vi "表格和打印表格.vi"() -> ()   [LabVIEW 2023]
panel:
  out "new picture":picture
  in  "Multicolumn Listbox":i32(listbox)
  # "表格以及打印表格"
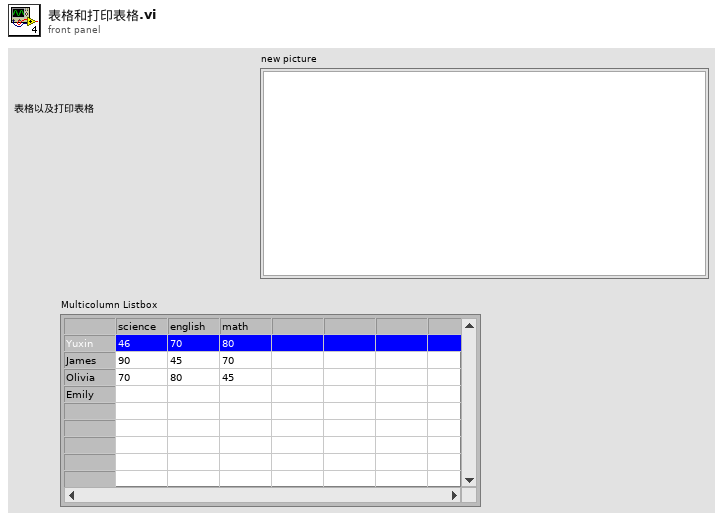
[diagram p1: front panel]
types:
  T1 = typedef "imagedata.ctl" = cluster{"image type":i32, "image depth":i32, "image":u8[], "mask":u8[], "colors":u32[], "Rectangle":cluster{"left":i16, "top":i16, "right":i16, "bottom":i16}}
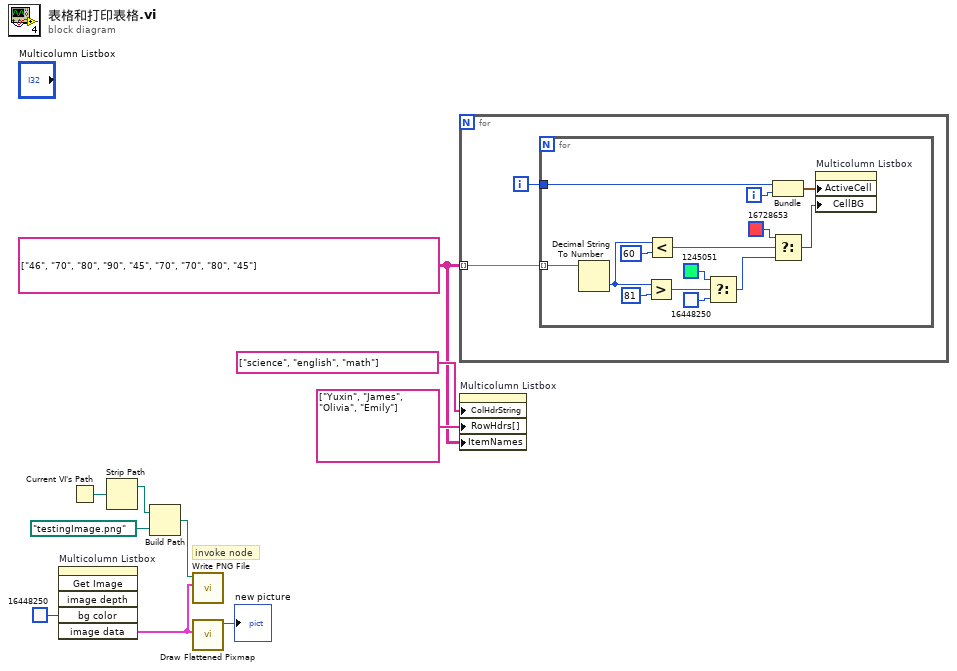
[diagram p0: block diagram]
diagram:
  w8 = string[][] [["46", "70", "80"], ["90", "45", "70"], ["70", "80", "45"]]
  # "invoke node"
  n1 = invoke on="Multicolumn Listbox" class="MCListbox (strict)" method="Get Image"("bg color"=u32 16448250) -> ("image data"=w5:T1)  [unwired: 5 in, 5 out]
  n2 = Current VI's Path() -> (path=w4:path)
  n3 = Strip Path(path=w4) -> (stripped path=w3:path)  [unwired: 1 out]
  n4 = Build Path(base path=w3, name or relative path=path "testingImage.png") -> (appended path=w1:path)
  n5 = call <vilib>:"Write PNG File.vi"("image data"=w5, "path to PNG file"=w1) -> ()  [unwired: 8 in, 2 out]
  n6 = call <vilib>:"Draw Flattened Pixmap.vi"("image data"=w5) -> ("new picture"=→"new picture":picture)  [unwired: 8 in]
  n7 = for {
    tunnel: w8 -> [w11] mode=indexing
    i -> [w12]
    n8 = for {
      tunnel: w12 -> [w26]
      tunnel: w11 -> [w23] mode=indexing
      i -> [w25]
      n9 = Decimal String To Number(string=w23) -> (number=w17:i32)  [unwired: 2 in, 1 out]
      n10 = Greater?(x=w17, y=81) -> (0:w15:bool)
      n11 = Less?(x=w17, y=60) -> (x < y?=w21:bool)
      n12 = Select(t=u32 1245051, s=w15, f=u32 16448250) -> (s? t:f=w18:u32)
      n13 = Bundle(w26, w25) -> (w24:cluster{i32, i32})  [unwired: 1 in]
      n14 = Select(t=u32 16728653, s=w21, f=w18) -> (s? t:f=w19:u32)
      n15 = property on="Multicolumn Listbox" class="MCListbox (strict)"("ActiveCell"=w24, "CellBG"=w19) -> ()  [unwired: 2 in, 2 out]
    }
  }
  n16 = property on="Multicolumn Listbox" class="MCListbox (strict)"("ColHdrString"=string[] ["science", "english", "math"], "RowHdrs[]"=string[] ["Yuxin", "James", "Olivia", "Emily"], "ItemNames"=w8) -> ()  [unwired: 2 in, 2 out]
